vi "Pre Launch Init.vi"(11 "Websocket Server in":refnum<class "Websocket Server.lvclass">) -> (0 "error out":errorcluster, 3 "Websocket Server out":refnum<class "Websocket Server.lvclass">)   [LabVIEW 2016, in "Stream Mediator.lvlib" / "Websocket Server.lvclass"]
doc: "--\nCopyright © 2017 Composed SystemsI All rights reserved.\n\nAuthor: Jon McBee <jon.mcbee@composed.io>\n\nThis library is provided \"AS IS\" ,WITHOUT WARRANTIES OR\nCONDITIONS OF ANY KIND, either express or implied.\n\nComposed Systems -- composed.io\n\nStream 0.0.1.1\nJon McBee - Composed Systems\nCopyright (c) 2017, Composed Systems"
uses:
  <userlib>/Composed Systems/Stream/Mediator/Classes/Websocket Server Actor/Websocket Server/Websocket Server.lvclass
  <userlib>/Composed Systems/Stream/Mediator/Classes/Subscriber Look Up Table/Subscriber Look Up Table.lvclass
  <userlib>/Composed Systems/Stream/Mediator/Classes/Websocket Server Actor/Websocket Server/Websocket Server.lvclass/Websocket Server.ctl
  <userlib>/Composed Systems/Stream/Mediator/Classes/Mediated Asynchronous Actor/Mediated Asynchronous Actor.lvclass
  <userlib>/Composed Systems/Stream/Look Up Table/Look Up Table/Look Up Table.lvclass
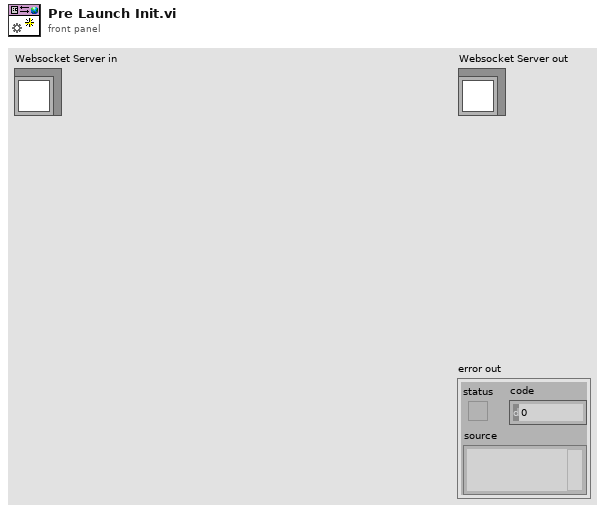
[diagram p1: front panel]
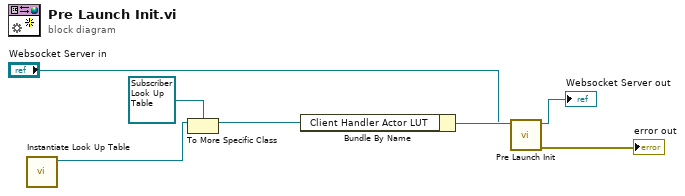
[diagram p0: block diagram]
diagram:
  n1 = call <userlib>:"Instantiate Look Up Table.vi"() -> ("Look Up Table out"=w4:refnum<class "Look Up Table.lvclass">)  [unwired: 10 in, 1 out]
  n2 = To More Specific Class(target class=refnum<class "Subscriber Look Up Table.lvclass"> refnum ("Stream Mediator.lvlib:Subscriber Look Up Table.lvclass"), reference=w4) -> (specific class reference=w3:refnum<class "Subscriber Look Up Table.lvclass">)  [unwired: 1 in, 1 out]
  n3 = Bundle By Name(cluster="Websocket Server in", "Client Handler Actor LUT"=w3) -> (w5:refnum<class "Websocket Server.lvclass">)
  n4 = call-parent "Pre Launch Init.vi"("Mediated Asynchronous Actor in"=w5) -> ("error out"=→"error out":errorcluster, "Mediated Asynchronous Actor out"=→"Websocket Server out":refnum<class "Websocket Server.lvclass">)  [unwired: 9 in]
